vi "ParseDataStorageSendData.vi"(8 "error in (no error)":errorcluster, 11 "body":variant) -> (0 "error out":errorcluster, 1 "block":i32, 2 "stream id":string, 3 "event reference":T1, 4 "properties":T2[](array[typedef]), 5 "DataEvent.Id":string)   [LabVIEW 2017]
uses:
  <vilib>/addons/InsightCM/MessageBus/Base/controls/KeyValuePair.ctl
  <vilib>/addons/InsightCM/Devices/Shared/Common/DataEvent/controls/EventReference.ctl
  <vilib>/addons/InsightCM/Devices/Shared/Common/DataEvent/controls/Event.ctl
  <vilib>/addons/InsightCM/MessageBus/Base/controls/DataEvent.ctl
  <vilib>/addons/InsightCM/Devices/Shared/Common/DataEvent/controls/DataSet.ctl
  <vilib>/addons/InsightCM/MessageBus/Base/controls/DataSetMetadata.ctl
  <vilib>/addons/InsightCM/MessageBus/Base/controls/TrendPoint.ctl
  <vilib>/addons/InsightCM/MessageBus/Base/controls/TrendAlarmUpdate.ctl
  <vilib>/addons/InsightCM/MessageBus/Base/controls/TrendAlarmTransition.ctl
  <vilib>/addons/InsightCM/Devices/Shared/Common/ServerComm/controls/SendDataEvent.ctl
  <vilib>/addons/InsightCM/Devices/Shared/Common/DataEvent/DataEvent.lvlib
  <vilib>/addons/InsightCM/Devices/Shared/Common/ServerComm/ServerComm.lvlib
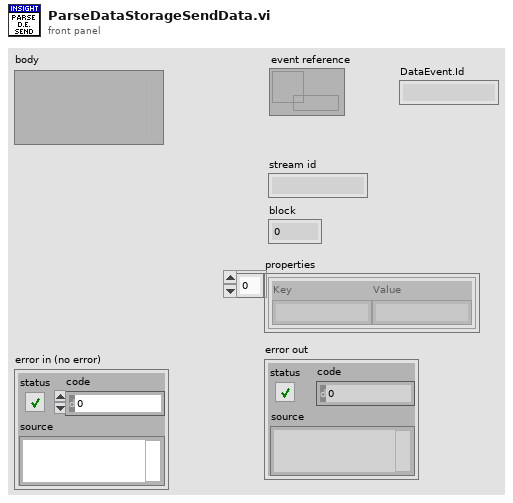
[diagram p1: front panel]
types:
  T1 = typedef "DataEvent.lvlib/EventReference.ctl" = refnum<data-value>
  T2 = typedef "KeyValuePair.ctl" = cluster{"Key":string, "Value":string}
  T3 = typedef "ServerComm.lvlib/SendDataEvent.ctl" = cluster{"event reference":T1, "StreamId":string, "Block":i32, "Properties":T2[]}
  T4 = typedef "DataEvent.lvlib/Event.ctl" = cluster{"DataEvent":T5, "DataSets":T6[], "TrendPoints":T8[], "Alarms":T9[]}
  T5 = typedef "DataEvent.ctl" = cluster{"Id":string, "AssetNodeId":string, "Timestamp":i64, "Props":T2[]}
  T6 = typedef "DataEvent.lvlib/DataSet.ctl" = cluster{"DataSetMetadata":T7, "Values":sgl[], "Values DVR":refnum<data-value>}
  T7 = typedef "DataSetMetadata.ctl" = cluster{"Id":string, "DataEventId":string, "AssetNodeId":string, "Type":string, "T0":i64, "Props":T2[]}
  T8 = typedef "TrendPoint.ctl" = cluster{"TrendPointId":string, "DataEventId":string, "Timestamp":i64, "Value":dbl, "Props":T2[]}
  T9 = typedef "TrendAlarmUpdate.ctl" = cluster{"RuleId":string, "Transition":T10}
  T10 = typedef "TrendAlarmTransition.ctl" = cluster{"At":i64, "Severity":i32, "Value":dbl}
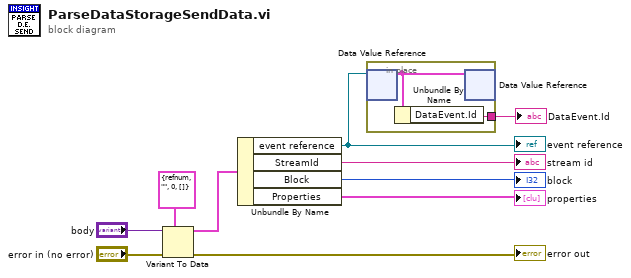
[diagram p0: block diagram]
diagram:
  n1 = Variant To Data(error in="error in (no error)", type=T3 {"event reference"=refnum, "StreamId"="", "Block"=0, "Properties"=[]} ("Body"), Variant="body") -> (data=w6:T3, error out=→"error out":errorcluster)
  n2 = Unbundle By Name(w6) -> ("event reference"=w2:T1, "StreamId"=→"stream id":string, "Block"=→"block":i32, "Properties"=→"properties":T2[])
  "event reference" <- w2
  n3 = in-place {
    in-place-border: [w11] -> w1
    n4 = in-place-dvr #1(w2) -> (w12:T4)  [unwired: 1 out]
    n5 = Unbundle By Name(w12) -> ("DataEvent.Id"=w11:string)
    n6 = in-place-dvr #1(w12) -> ()  [unwired: 2 out]
  }
  "DataEvent.Id" <- w1
